vi "HEWH Select Unit Type.vi"(8 "error in (no error)":errorcluster) -> (0 "error out":errorcluster, 3 "Unit Type":string(combo))   [LabVIEW 2016]
uses:
  Utility/Custom Pallet Controls/Custom Pallet Forward.ctl
panel:
  in  "Tab Control":enum32{"Page 1", "Page 2"}(tab)
  out "Description":string="Select Unit Type"
  in  "80 Gallon":bool
  in  "50 Gallon":bool
  in  "File Setup OK":T1
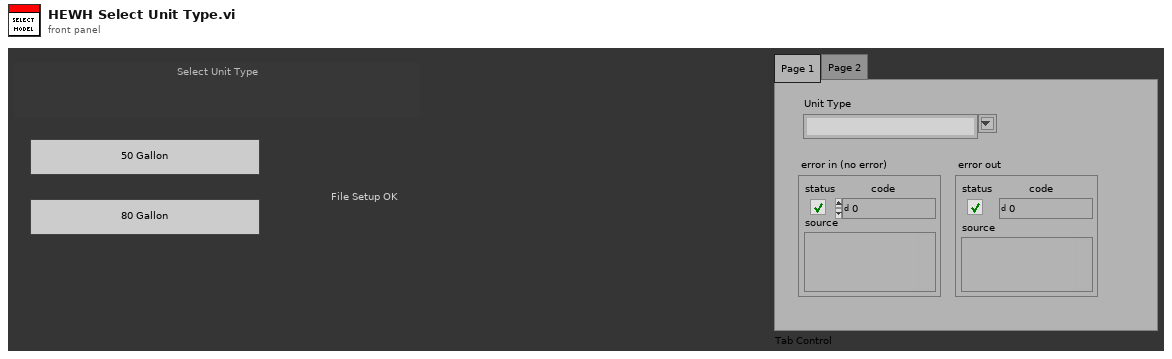
[diagram p1: front panel]
types:
  T1 = typedef "Custom Pallet Forward.ctl" = bool
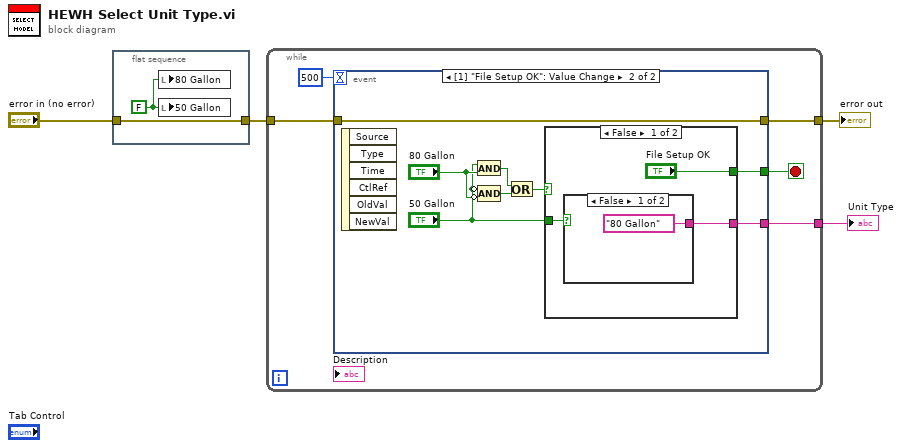
[diagram p0: block diagram]
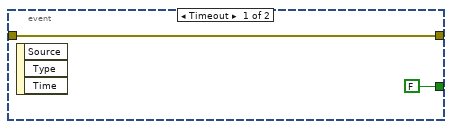
[diagram p2: hidden frame]
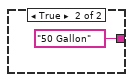
[diagram p3: hidden frame]
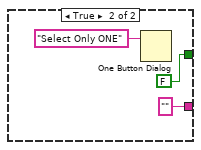
[diagram p4: hidden frame]
diagram:
  n1 = flat-sequence {
    tunnel: "error in (no error)" -> [w6]
    tunnel: [w6] -> w1
    frame #0 {
      w5 = FALSE ("80 Gallon")
      n2 = local write "80 Gallon"(w5) -> ()
      n3 = local write "50 Gallon"(w5) -> ()
    }
  }
  n4 = while {
    tunnel: [w11] -> w4
    tunnel: w1 -> [w9]
    tunnel: [w8] -> w3
    stop <- w10 stop-if-true
    n5 = event shown="[1] \"File Setup OK\": Value Change" {
      selector: _ -> [_ _]
      dyn-events: _ -> [_ _]
      timeout: 500 -> [_ _]
      tunnel: [_ w21] -> w11
      tunnel: [T1 FALSE ("File Setup OK") w20] -> w10
      tunnel: [w13 w14] -> w8
      tunnel: w9 -> [w13 w14]
      event Timeout {
        n6 = event-data() -> ()  [unwired: 1 in, 3 out]
      }
      event Value Change {
        n7 = event-data() -> ()  [unwired: 1 in, 6 out]
        n8 = And(x="50 Gallon", y="80 Gallon") -> (x .and. y?=w15:bool)
        n9 = Compound Arithmetic op=AND(invert "50 Gallon", invert "80 Gallon") -> (w16:bool)
        n10 = Or(x=w15, y=w16) -> (x .or. y?=w19:bool)
        n11 = case shown="False" w19 {
          tunnel: ["File Setup OK" T1 FALSE ("File Setup OK")] -> w20
          tunnel: "50 Gallon" -> [w23 _]
          tunnel: [w22 "" ("Unit Type")] -> w21
          frame False {
            n12 = case shown="False" w23 {
              tunnel: ["80 Gallon" ("Unit Type") "50 Gallon" ("Unit Type")] -> w22
              frame False {
              }
              frame True {
              }
            }
          }
          frame True {
            n13 = One Button Dialog(message="Select Only ONE") -> ()  [unwired: 1 in, 1 out]
          }
        }
      }
    }
  }
  "Unit Type" <- w4
  "error out" <- w3
